vi "test Get Status Channel Error References.vi"(8 "error in":errorcluster, 11 "TestCase in":refnum<class "Scripting.lvclass">) -> (0 "error out":errorcluster, 3 "TestCase out":refnum<class "Scripting.lvclass">)   [LabVIEW 2020, in "Scripting.lvclass"]
uses:
  Scripting.lvclass
  <vilib>/addons/_JKI Toolkits/VI Tester/TestCase.llb/TestCase.lvclass
  Scripting/Ballard ARINC 429 Scripting.lvlib
  <vilib>/NI VeriStand/Custom Device API/Custom Device Item Ref.ctl
  <vilib>/NI VeriStand/Custom Device API/Custom Device API.lvlib
  C:/Program Files (x86)/National Instruments/LabVIEW 2020/vi.lib/addons/_JKI Toolkits/VI Tester/TestCase.llb/TestCase.lvclass
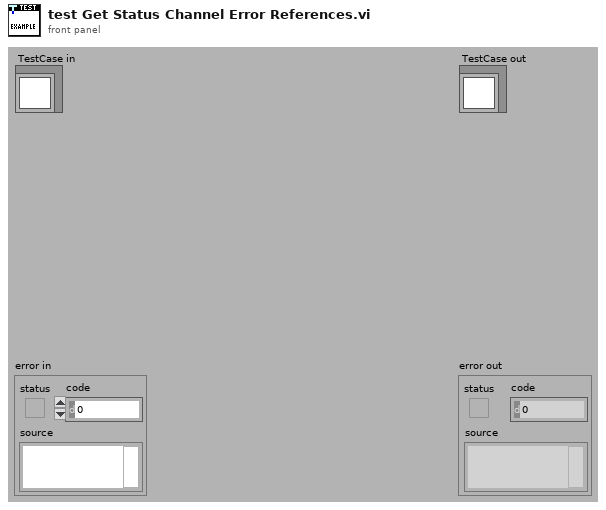
[diagram p1: front panel]
types:
  T1 = typedef "Custom Device API.lvlib/Custom Device Item Ref.ctl" = u64
  T2 = cluster{"gap":T1, "parity":T1, "long word":T1, "bit timing":T1, "timeout":T1}
  T3 = cluster{"gap":bool, "parity":bool, "long word":bool, "bit timing":bool, "timeout":bool}
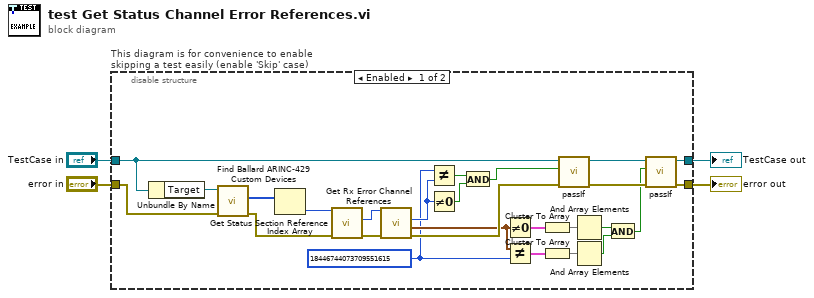
[diagram p0: block diagram]
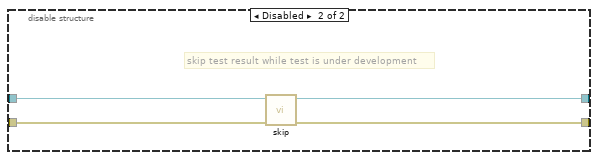
[diagram p2: hidden frame]
diagram:
  n1 = disable-structure "This diagram is for convenience to enable skipping a test easily (enable 'Skip' case)" shown="Enabled" {
    disable-tunnel: "TestCase in" -> [w29 w34]
    disable-tunnel: [w28 w32] -> w1
    disable-tunnel: [w25 w33] -> w3
    disable-tunnel: "error in" -> [w26 w31]
    frame Enabled {
      w11 = T1 18446744073709551615 ("Rx error count reference")
      n2 = Unbundle By Name(w29) -> ("Target"=w30:refnum<k24>)
      n3 = call "Find Ballard ARINC-429 Custom Devices.vi"("error in"=w26, "target in"=w30) -> ("error out"=w23:errorcluster, "Ballard ARINC 429 custom devices"=w5:u64[])  [unwired: 7 in, 1 out]
      n4 = Index Array(array=w5) -> (element=w24:u64)  [unwired: 1 in]
      n5 = call "Get Status Section Reference.vi"("error in"=w23, "Ballard ARINC 429 ref"=w24) -> ("error out"=w21:errorcluster, "status section reference"=w22:T1)  [unwired: 7 in, 1 out]
      n6 = call "Get Rx Error Channel References.vi"("error in"=w21, "status reference in"=w22) -> ("error out"=w17:errorcluster, "Rx specific error count references"=w12:T2, "Rx error count reference"=w16:T1)  [unwired: 6 in, 1 out]
      n7 = Not Equal?(x=w11, y=w16) -> (x != y?=w15:bool)
      n8 = Not Equal To 0?(x=w16) -> (x != 0?=w14:bool)
      n9 = And(x=w15, y=w14) -> (x .and. y?=w13:bool)
      n10 = Not Equal To 0?(x=w12) -> (x != 0?=w20:cluster{bool, bool, bool, bool, bool})
      n11 = Not Equal?(x=w12, y=w11) -> (x != y?=w10:T3)
      n12 = Cluster To Array(cluster=w20) -> (array=w19:bool[])
      n13 = Cluster To Array(cluster=w10) -> (array=w9:bool[])
      n14 = call-dynamic "passIf.vi"("error in (no error)"=w17, "pass"=w13, "TestCase in"=w29) -> ("error out"=w18:errorcluster, "TestCase out"=w27:refnum<class "Scripting.lvclass">)  [unwired: 7 in]
      n15 = And Array Elements(Boolean array=w19) -> (logical AND=w8:bool)
      n16 = And Array Elements(Boolean array=w9) -> (logical AND=w7:bool)
      n17 = And(x=w8, y=w7) -> (x .and. y?=w6:bool)
      n18 = call-dynamic "passIf.vi"("error in (no error)"=w18, "pass"=w6, "TestCase in"=w27) -> ("error out"=w25:errorcluster, "TestCase out"=w28:refnum<class "Scripting.lvclass">)  [unwired: 7 in]
    }
    frame Disabled {
      # "skip test result while test is under development"
      n19 = call <vilib>:"skip.vi"("error in (no error)"=w31, "TestCase in"=w34) -> ("error out"=w33:errorcluster, "TestCase out"=w32:refnum<class "Scripting.lvclass">)  [unwired: 8 in]
    }
  }
  "error out" <- w3
  "TestCase out" <- w1
